vi "State Machine.vi"   [LabVIEW 2020]
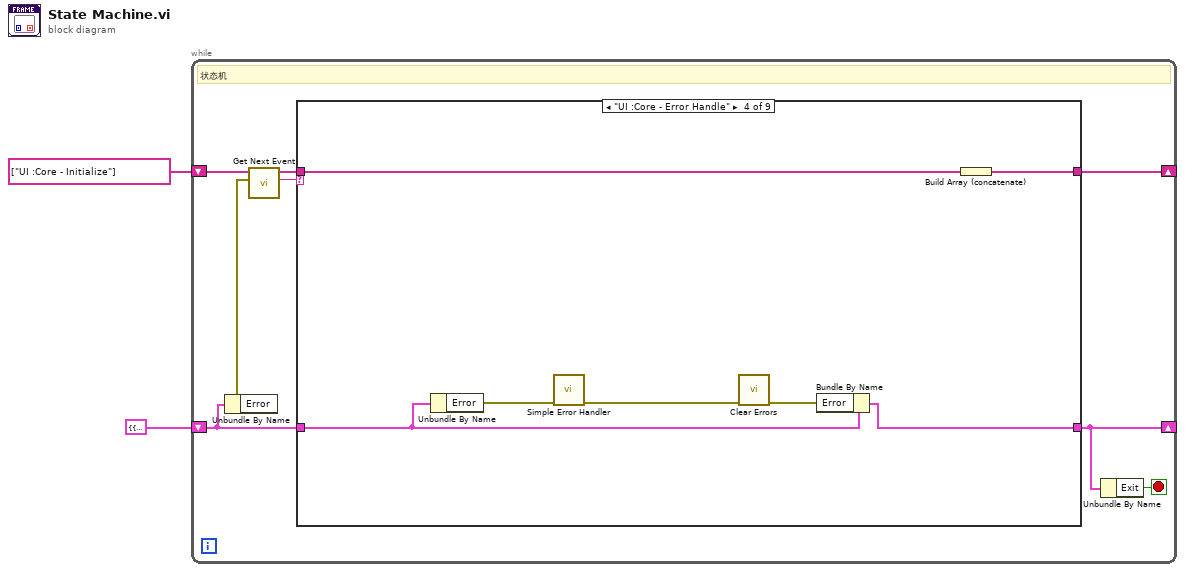
[diagram p0: block diagram]
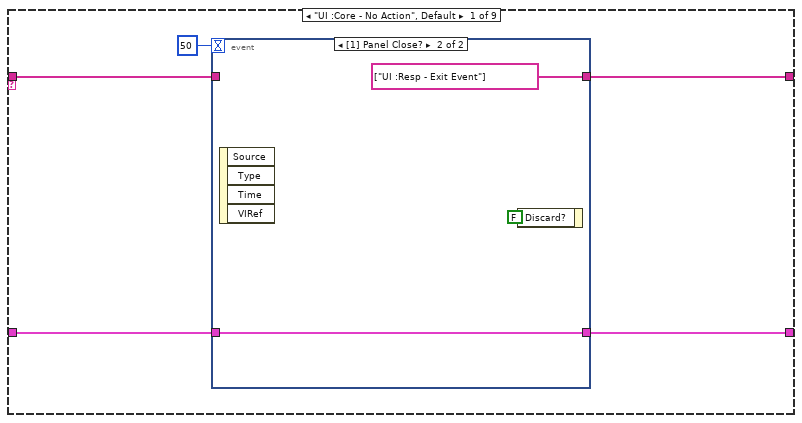
[diagram p2: hidden frame]
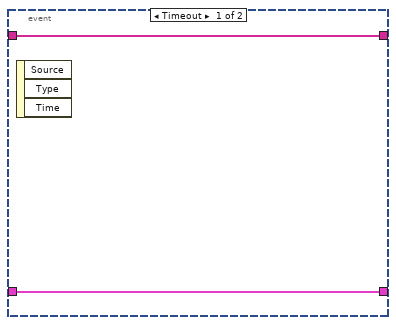
[diagram p3: hidden frame]
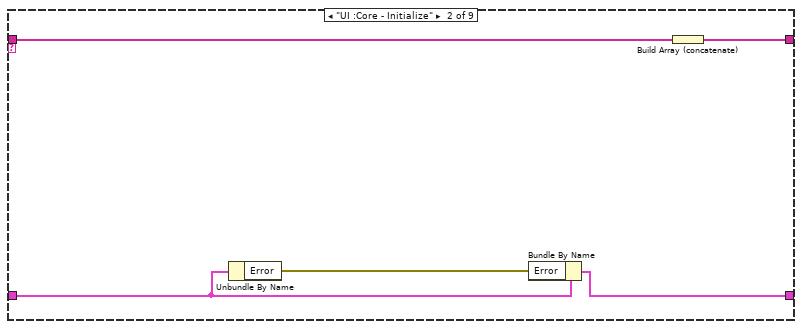
[diagram p4: hidden frame]
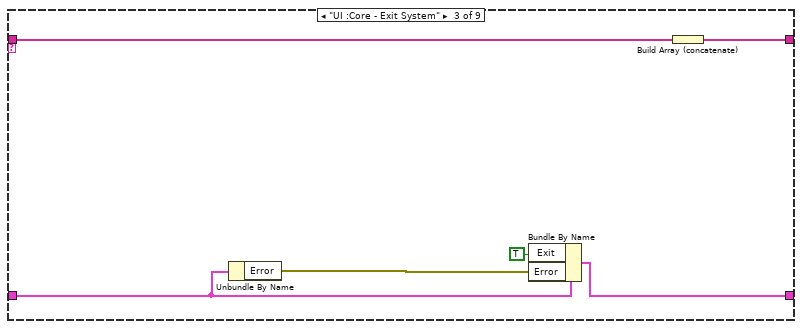
[diagram p5: hidden frame]
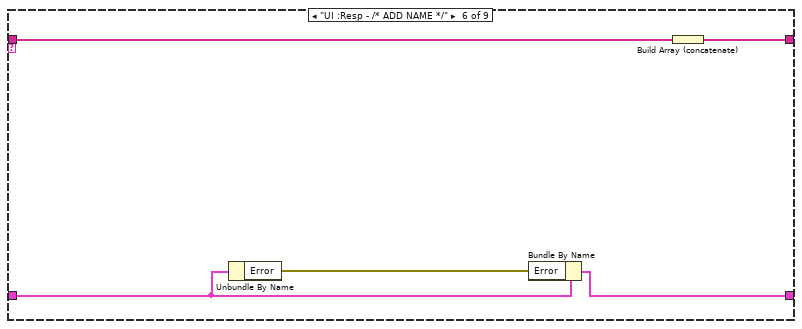
[diagram p7: hidden frame]
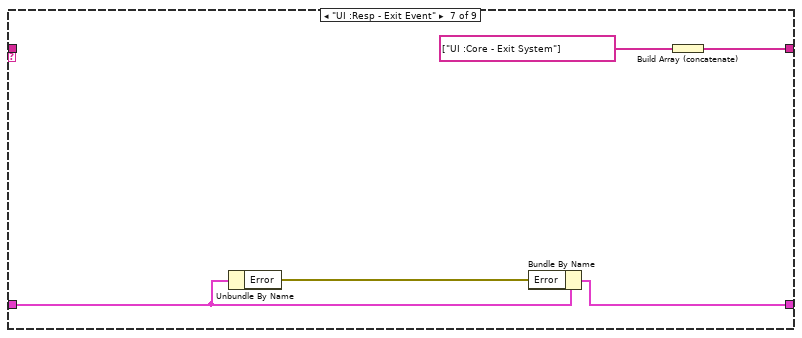
[diagram p8: hidden frame]
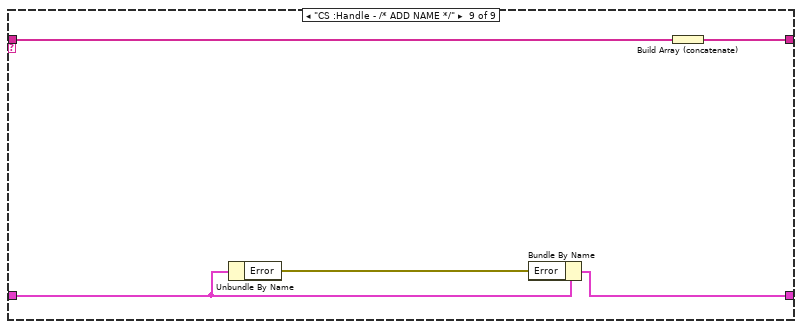
[diagram p10: hidden frame]
diagram:
  n1 = while {
    shift-right: [w5] -> _
    shift-left: string[] ["UI :Core - Initialize"] -> [w8]
    shift-right: [w4] -> _
    shift-left: cluster{"Error":errorcluster, "Exit":bool} {"Error"={"status"=FALSE, "code"=0, "source"=""}, "Exit"=FALSE} ("Temp Variable") -> [w7]
    stop <- w3 stop-if-true
    # "状态机"
    n2 = Unbundle By Name(w7) -> ("Error"=w6:errorcluster)
    n3 = call "Get Next Event.vi"("error in (no error)"=w6, "event queue in"=w8) -> ("next event"=w9:string, "event queue out"=w10:string[])  [unwired: 8 in]
    n4 = case shown="\"UI :Core - Error Handle\"" w9 {
      tunnel: w10 -> [w12 w25 w31 w38 w40 w45 _ w51 w57]
      tunnel: w7 -> [w14 w23 w29 w36 w39 w43 w49 w52 w55]
      tunnel: [w11 w24 w30 w37 w40 w44 w50 w51 w56] -> w5
      tunnel: [w13 w21 w28 w35 w39 w42 w48 w52 w54] -> w4
      frame "UI :Core - No Action", Default {
        n5 = event shown="[1] Panel Close?" {
          selector: _ -> [_ _]
          dyn-events: _ -> [_ _]
          timeout: 50 -> [_ _]
          tunnel: w14 -> [w17 w20]
          tunnel: [w17 w20] -> w13
          tunnel: w12 -> [w16 _]
          tunnel: [w16 string[] ["UI :Resp - Exit Event"] ("event queue out")] -> w11
          event Timeout {
            n6 = event-data() -> ()  [unwired: 1 in, 3 out]
          }
          event Panel Close? {
            n7 = event-data() -> ()  [unwired: 1 in, 4 out]
            n8 = event-data("Discard?"=FALSE) -> ()  [unwired: 1 in, 1 out]
          }
        }
      }
      frame "UI :Core - Initialize" {
        n9 = Unbundle By Name(w23) -> ("Error"=w22:errorcluster)
        n10 = Bundle By Name(cluster=w23, "Error"=w22) -> (w21:cluster{"Error":errorcluster, "Exit":bool})
        n11 = Build Array (concatenate)(w25) -> (w24:string[])
      }
      frame "UI :Core - Exit System" {
        n12 = Unbundle By Name(w29) -> ("Error"=w27:errorcluster)
        n13 = Bundle By Name(cluster=w29, "Exit"=TRUE, "Error"=w27) -> (w28:cluster{"Error":errorcluster, "Exit":bool})
        n14 = Build Array (concatenate)(w31) -> (w30:string[])
      }
      frame "UI :Core - Error Handle" {
        n15 = Unbundle By Name(w36) -> ("Error"=w34:errorcluster)
        n16 = call <vilib>:"Simple Error Handler.vi"("error in (no error)"=w34) -> ("error out"=w32:errorcluster)  [unwired: 4 in, 4 out]
        n17 = call <vilib>:"Clear Errors.vi"("error in (no error)"=w32) -> ("error out"=w33:errorcluster)  [unwired: 5 in, 1 out]
        n18 = Bundle By Name(cluster=w36, "Error"=w33) -> (w35:cluster{"Error":errorcluster, "Exit":bool})
        n19 = Build Array (concatenate)(w38) -> (w37:string[])
      }
      frame "---------------------------------UI :Resp---------------------------------" {
      }
      frame "UI :Resp - /* ADD NAME */" {
        n20 = Unbundle By Name(w43) -> ("Error"=w41:errorcluster)
        n21 = Bundle By Name(cluster=w43, "Error"=w41) -> (w42:cluster{"Error":errorcluster, "Exit":bool})
        n22 = Build Array (concatenate)(w45) -> (w44:string[])
      }
      frame "UI :Resp - Exit Event" {
        n23 = Unbundle By Name(w49) -> ("Error"=w47:errorcluster)
        n24 = Bundle By Name(cluster=w49, "Error"=w47) -> (w48:cluster{"Error":errorcluster, "Exit":bool})
        n25 = Build Array (concatenate)(string[] ["UI :Core - Exit System"] ("event queue out")) -> (w50:string[])
      }
      frame "--------------------------------CS :Handle-------------------------------" {
      }
      frame "CS :Handle - /* ADD NAME */" {
        n26 = Unbundle By Name(w55) -> ("Error"=w53:errorcluster)
        n27 = Bundle By Name(cluster=w55, "Error"=w53) -> (w54:cluster{"Error":errorcluster, "Exit":bool})
        n28 = Build Array (concatenate)(w57) -> (w56:string[])
      }
    }
    n29 = Unbundle By Name(w4) -> ("Exit"=w3:bool)
  }
